vi "ReadHemisphereData.vi"(8 "Error in":errorcluster, 10 "Hemisphere Queue Cluster":T1, 11 "VISA UART port":refnum<visa-resource-name>) -> (0 "Error out":errorcluster)   [LabVIEW 2013]
uses:
  Data/TypeDefs/UTM Location.ctl
  Data/TypeDefs/GPS Sensor Status.ctl
  Data/TypeDefs/GPS-Compass Queue Cluster.ctl
panel:
  out "Longitude [deg]":string
  out "Latitude [deg]":string
  in  "time zone":i32
  out "Time":string
  out "Mode":string
  out "Date [ddmmyy]":string
  out "Course over ground [degrees]":string
  out "Status":string
  out "Speed over ground [knots]":string
  out "E/W":string
  out "Longitude":string
  out "N/S":string
  out "Latitude":string
  out "UTC Time":string
  out "1PPS":bool
  out "NMEA sentences":string
  # "GPS demo"
  # "[hhmmss.sss]"
  # "A = vAlid data\nV = inValid data"
  # "[ddmm.mmmm]"
  # "[dddmm.mmmm]"
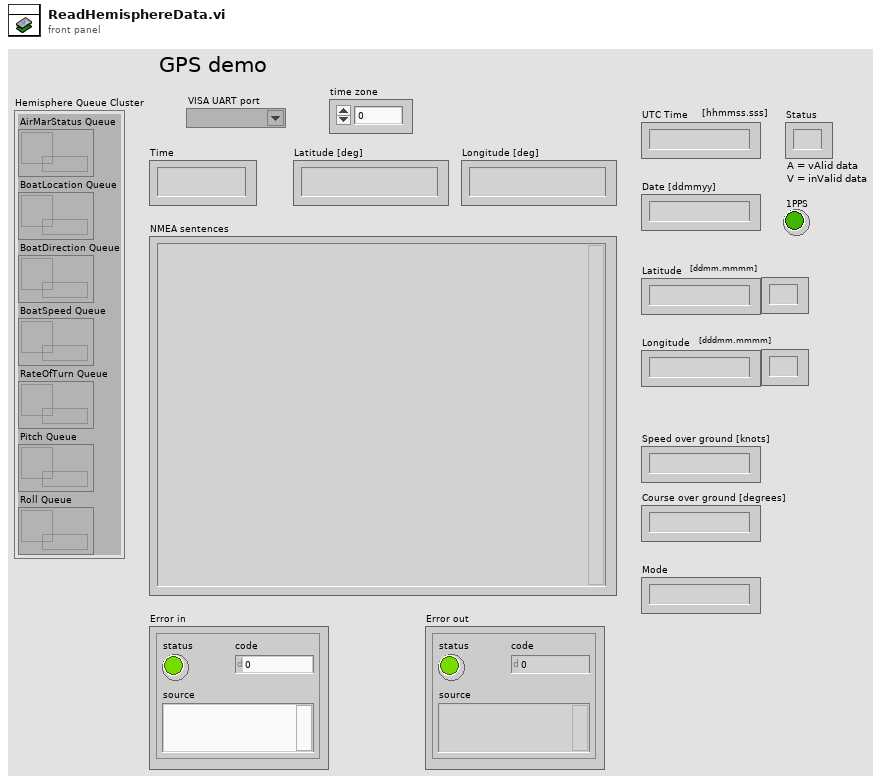
[diagram p1: front panel]
types:
  T1 = typedef "GPS-Compass Queue Cluster.ctl" = cluster{"AirMarStatus Queue":refnum<queue>, "BoatLocation Queue":refnum<queue>, "BoatDirection Queue":refnum<queue>, "BoatSpeed Queue":refnum<queue>, "RateOfTurn Queue":refnum<queue>, "Pitch Queue":refnum<queue>, "Roll Queue":refnum<queue>}
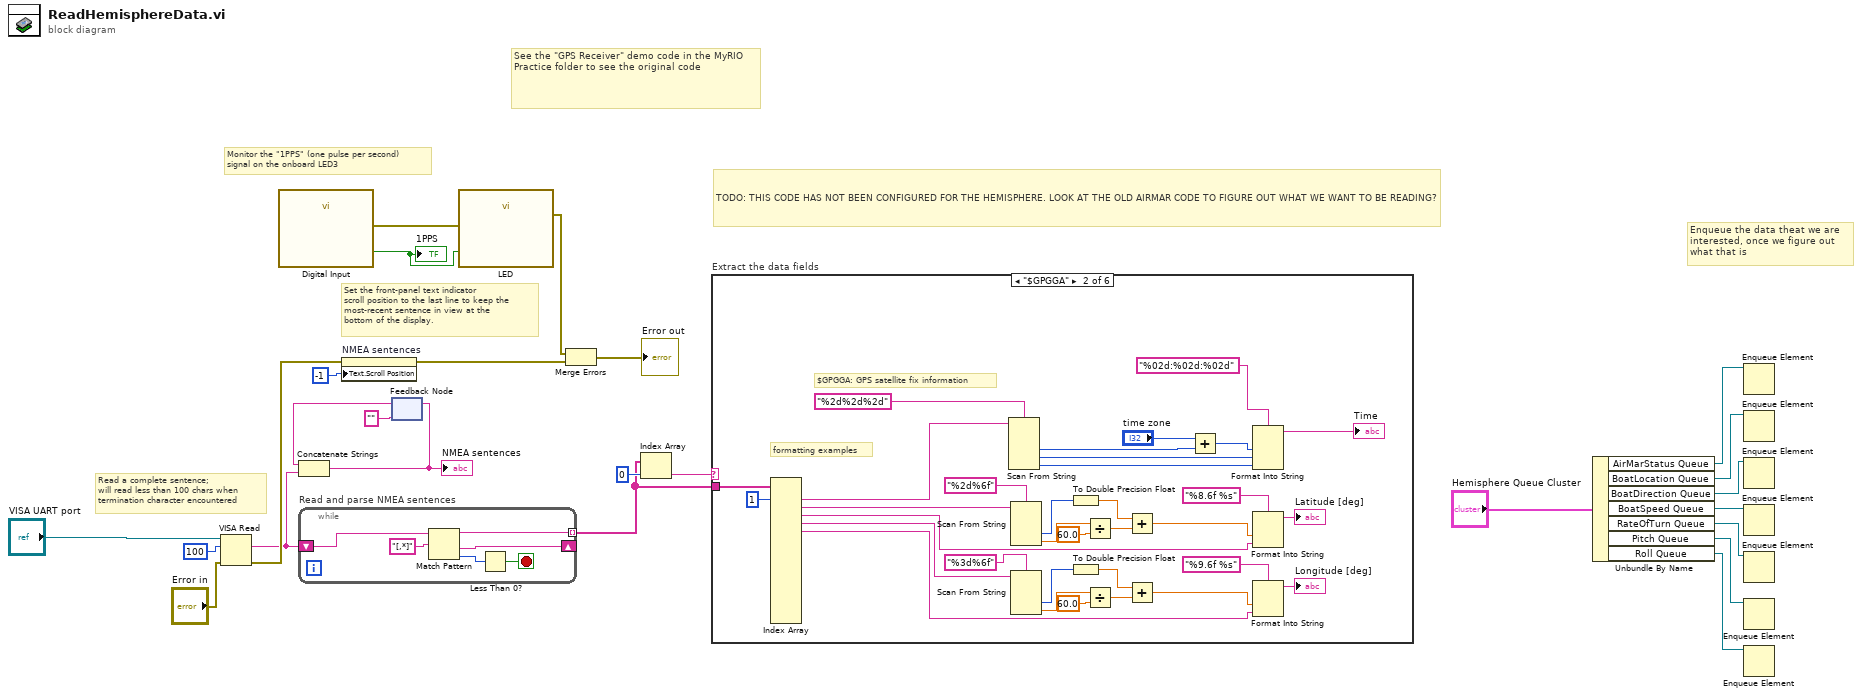
[diagram p0: block diagram]
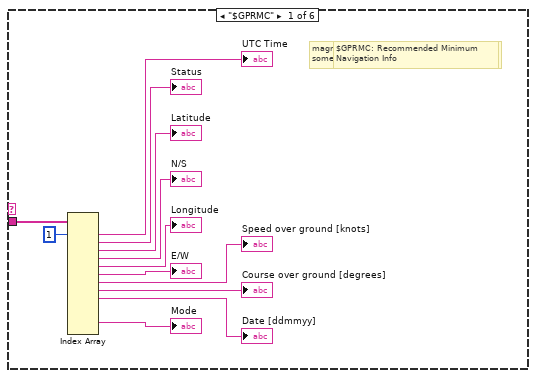
[diagram p2: hidden frame]
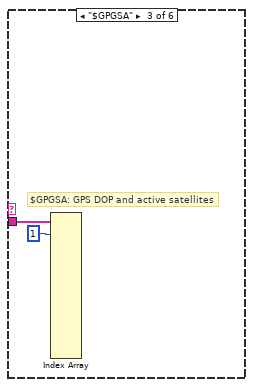
[diagram p3: hidden frame]
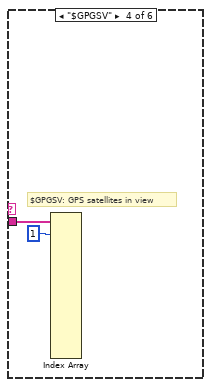
[diagram p4: hidden frame]
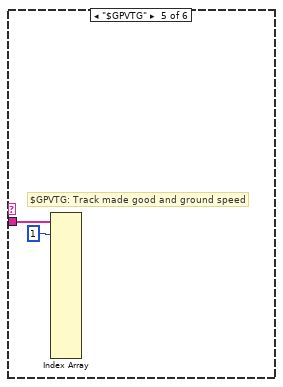
[diagram p5: hidden frame]
diagram:
  # "Enqueue the data theat we are interested, once we figure out what that is"
  # "TODO: THIS CODE HAS NOT BEEN CONFIGURED FOR THE HEMISPHERE. LOOK AT THE OLD AIRMAR CODE TO FIGURE OUT WHAT WE WANT TO BE READING?"
  # "Set the front-panel text indicator\nscroll position to the last line to keep the\nmost-recent sentence in view at the\nbottom of the display."
  # "Read a complete sentence;\nwill read less than 100 chars when\ntermination character encountered"
  # "Monitor the \"1PPS\" (one pulse per second)\nsignal on the onboard LED3"
  # "See the \"GPS Receiver\" demo code in the MyRIO Practice folder to see the original code"
  n1 = VISA Read(VISA resource name="VISA UART port", byte count=u32 100, error in (no error)="Error in") -> (read buffer=w16:string, error out=w21:errorcluster)  [unwired: 2 out]
  n2 = call "Digital Input"() -> ("A/DIO0 (Pin 11)"=w23:bool, "error out"=w24:errorcluster)  [unwired: 26 in]
  "1PPS" <- w23
  n3 = while "Read and parse NMEA sentences" {
    tunnel: [w29] -> w18 mode=indexing
    shift-right: [w28] -> _
    shift-left: w16 -> [w30]
    stop <- w27 stop-if-true
    n4 = Match Pattern(string=w30, regular expression="[,*]") -> (before substring=w29:string, after substring=w28:string, offset past match=w26:i32)  [unwired: 1 in, 1 out]
    n5 = Less Than 0?(x=w26) -> (x < 0?=w27:bool)
  }
  n6 = property on="NMEA sentences" class="Str"(error in=w21, "Text.Scroll Position"=-1) -> (error out=w9:errorcluster)  [unwired: 1 in, 1 out]
  n7 = feedback #1("") -> (w14:string)
  n8 = Concatenate Strings "Concatenate Strings"(w14, w16) -> (w12:string)
  "NMEA sentences" <- w12
  n9 = feedback-in #1(w12) -> ()
  n10 = call "LED"("LED3"=w23, "error in (no error)"=w24) -> ("error out"=w22:errorcluster)  [unwired: 25 in]
  n11 = Merge Errors "Merge Errors"(w22, w9) -> (→"Error out":errorcluster)
  n12 = Index Array "Index Array"(array=w18, index=0) -> (element=w17:string)
  n13 = case "Extract the data fields" shown="\"$GPGGA\"" w17 {
    tunnel: w18 -> [w43 w76 w78 w80 w82 _]
    frame "$GPRMC" {
      # "magnetic variation not available w/o\nsome firmware upgrade from GlobalTop"
      # "$GPRMC: Recommended Minimum\nNavigation Info"
      n14 = Index Array "Index Array"(array=w43, index #1=1 ("index")) -> (element #1=→"UTC Time":string, element #2=→"Status":string, element #3=→"Latitude":string, element #4=→"N/S":string, element #5=→"Longitude":string, element #6=→"E/W":string, element #7=→"Speed over ground [knots]":string, element #8=→"Course over ground [degrees]":string, element #9=→"Date [ddmmyy]":string, element #12=→"Mode":string)  [unwired: 12 in, 3 out]
    }
    frame "$GPGGA" {
      # "formatting examples"
      # "$GPGGA: GPS satellite fix information"
      n15 = Index Array "Index Array"(array=w76, index #1=1 ("index")) -> (element #1=w73:string, element #2=w64:string, element #3=w56:string, element #4=w45:string, element #5=w44:string)  [unwired: 15 in, 11 out]
      n16 = Scan From String "Scan From String"(format string="%2d%2d%2d", input string=w73) -> (output 1=w66:i32, output 2=w69:i32, output 3=w71:i32)  [unwired: 5 in, 3 out]
      n17 = Scan From String(format string="%2d%6f", input string=w64) -> (output 1=w61:i32, output 2=w63:dbl)  [unwired: 4 in, 3 out]
      n18 = Scan From String(format string="%3d%6f", input string=w45) -> (output 1=w49:i32, output 2=w47:dbl)  [unwired: 4 in, 3 out]
      n19 = To Double Precision Float(number=w61) -> (double precision float=w59:dbl)
      n20 = To Double Precision Float(number=w49) -> (double precision float=w51:dbl)
      n21 = Divide(x=w63, y=60.0) -> (x/y=w60:dbl)
      n22 = Divide(x=w47, y=60.0) -> (x/y=w50:dbl)
      n23 = Add(x=w59, y=w60) -> (x+y=w57:dbl)
      n24 = Add(x=w51, y=w50) -> (x+y=w53:dbl)
      n25 = Add(x="time zone", y=w66) -> (x+y=w67:i32)
      n26 = Format Into String "Format Into String"(format string="%02d:%02d:%02d", w67, w69, w71) -> (resulting string=→"Time":string)  [unwired: 2 in, 1 out]
      n27 = Format Into String(format string="%8.6f %s", w57, w56) -> (resulting string=→"Latitude [deg]":string)  [unwired: 2 in, 1 out]
      n28 = Format Into String(format string="%9.6f %s", w53, w44) -> (resulting string=→"Longitude [deg]":string)  [unwired: 2 in, 1 out]
    }
    frame "$GPGSA" {
      # "$GPGSA: GPS DOP and active satellites"
      n29 = Index Array(array=w78, index #1=1 ("index")) -> ()  [unwired: 15 in, 16 out]
    }
    frame "$GPGSV" {
      # "$GPGSV: GPS satellites in view"
      n30 = Index Array(array=w80, index #1=1 ("index")) -> ()  [unwired: 15 in, 16 out]
    }
    frame "$GPVTG" {
      # "$GPVTG: Track made good and ground speed"
      n31 = Index Array(array=w82, index #1=1 ("index")) -> ()  [unwired: 15 in, 16 out]
    }
    frame Default {
    }
  }
  n32 = Unbundle By Name("Hemisphere Queue Cluster") -> ("AirMarStatus Queue"=w7:refnum<queue>, "BoatLocation Queue"=w6:refnum<queue>, "BoatDirection Queue"=w5:refnum<queue>, "BoatSpeed Queue"=w4:refnum<queue>, "RateOfTurn Queue"=w3:refnum<queue>, "Pitch Queue"=w2:refnum<queue>, "Roll Queue"=w1:refnum<queue>)
  n33 = Enqueue Element(queue=w7) -> ()  [unwired: 3 in, 3 out]
  n34 = Enqueue Element(queue=w6) -> ()  [unwired: 3 in, 3 out]
  n35 = Enqueue Element(queue=w5) -> ()  [unwired: 3 in, 3 out]
  n36 = Enqueue Element(queue=w4) -> ()  [unwired: 3 in, 3 out]
  n37 = Enqueue Element(queue=w3) -> ()  [unwired: 3 in, 3 out]
  n38 = Enqueue Element(queue=w2) -> ()  [unwired: 3 in, 3 out]
  n39 = Enqueue Element(queue=w1) -> ()  [unwired: 3 in, 3 out]
